vi "myRIO_BRig_RT__Case_Exp_subState_LC__ENL2.vi"(7 "input_spout":enum16{"Left", "Right"}(ring), 8 "input_dataCurrent":u16[](array[numeric]), 10 "input_dataLC":u16[](array[numeric])) -> (2 "output_LC":bool)   [LabVIEW 2014]
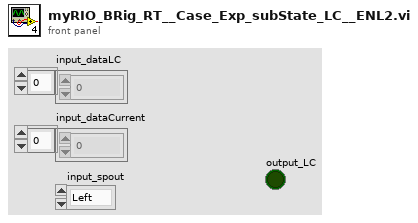
[diagram p1: front panel]
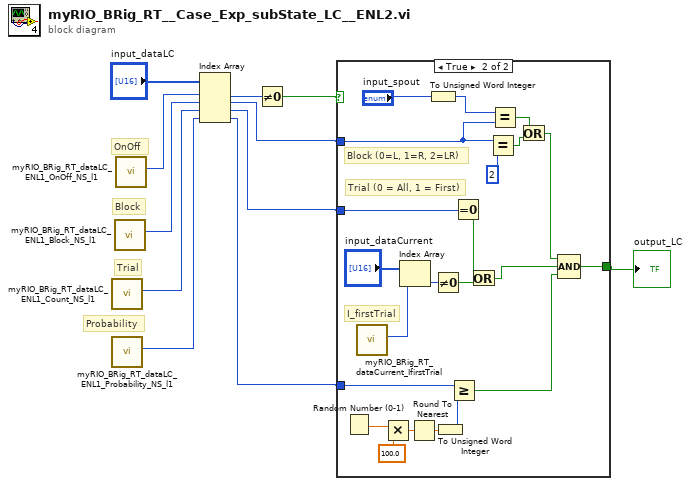
[diagram p0: block diagram]
diagram:
  # "Probability"
  # "Trial"
  # "Block"
  # "OnOff"
  n1 = call "myRIO_BRig_RT_dataLC_ENL1_Count_NS_l1.vi"() -> ("output_ENL1_Count_NS_l1"=w8:i32)  [unwired: 11 in]
  n2 = call "myRIO_BRig_RT_dataLC_ENL1_Probability_NS_l1.vi"() -> ("output_ENL1_Probability_NS_l1"=w7:i32)  [unwired: 11 in]
  n3 = call "myRIO_BRig_RT_dataLC_ENL1_Block_NS_l1.vi"() -> ("output_ENL1_All_Block"=w9:i32)  [unwired: 11 in]
  n4 = call "myRIO_BRig_RT_dataLC_ENL1_OnOff_NS_l1.vi"() -> ("output_ENL1_OnOff_NS_l1"=w10:i32)  [unwired: 11 in]
  n5 = Index Array(array="input_dataLC", index #1=w10, index #2=w9, index #3=w8, index #4=w7) -> (element #1=w6:u16, element #2=w4:u16, element #3=w3:u16, element #4=w2:u16)
  n6 = Not Equal To 0?(x=w6) -> (x != 0?=w5:bool)
  n7 = case shown="True" w5 {
    tunnel: [_ w21] -> w1
    tunnel: w4 -> [_ w14]
    tunnel: w3 -> [_ w17]
    tunnel: w2 -> [_ w18]
    frame False {
    }
    frame True {
      # "Block (0=L, 1=R, 2=LR)"
      # "Trial (0 = All, 1 = First)"
      # "I_firstTrial"
      n8 = Random Number (0-1)() -> (number: 0 to 1=w26:dbl)
      n9 = call "myRIO_BRig_RT_dataCurrent_IfirstTrial.vi"() -> ("output_I_firstTrial"=w30:i32)  [unwired: 11 in]
      n10 = Multiply(x=w26, y=100.0) -> (x*y=w25:dbl)
      n11 = Index Array(array="input_dataCurrent", index=w30) -> (element=w29:u16)
      n12 = Round To Nearest(number=w25) -> (nearest integer value=w24:dbl)
      n13 = To Unsigned Word Integer(number="input_spout") -> (unsigned 16bit integer=w13:u16)
      n14 = Not Equal To 0?(x=w29) -> (x != 0?=w27:bool)
      n15 = To Unsigned Word Integer(number=w24) -> (unsigned 16bit integer=w23:u16)
      n16 = Greater Or Equal?(x=w18, y=w23) -> (x >= y?=w12:bool)
      n17 = Equal To 0?(x=w17) -> (x = 0?=w28:bool)
      n18 = Or(x=w28, y=w27) -> (x .or. y?=w16:bool)
      n19 = Equal?(x=w14, y=u16 2) -> (x = y?=w31:bool)
      n20 = Equal?(x=w13, y=w14) -> (x = y?=w32:bool)
      n21 = Or(x=w32, y=w31) -> (x .or. y?=w15:bool)
      n22 = Compound Arithmetic op=AND(w15, w16, w12) -> (w21:bool)
    }
  }
  "output_LC" <- w1
